vi "Calculate Best Angle.vi"(8 "Bearing Clearence":dbl, 9 "Desired Bearing":dbl, 10 "Angle (max)":dbl, 11 "Angle (min)":dbl) -> (3 "Command Heading":dbl)   [LabVIEW 2011]
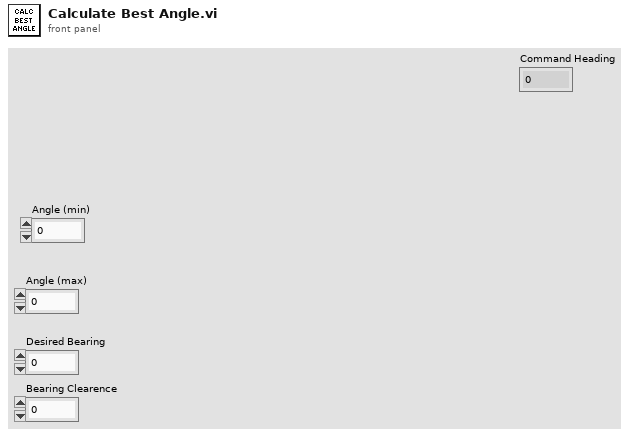
[diagram p1: front panel]
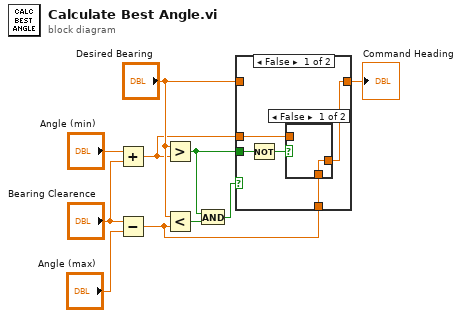
[diagram p0: block diagram]
diagram:
  n1 = Add(x="Angle (min)", y="Bearing Clearence") -> (x+y=w2:dbl)
  n2 = Subtract(x="Bearing Clearence", y="Angle (max)") -> (x-y=w1:dbl)
  n3 = Greater?(x="Desired Bearing", y=w2) -> (0:w3:bool)
  n4 = Less?(x="Desired Bearing", y=w1) -> (x < y?=w7:bool)
  n5 = And(x=w3, y=w7) -> (x .and. y?=w6:bool)
  n6 = case shown="False" w6 {
    tunnel: "Desired Bearing" -> [_ w18]
    tunnel: [w12 w18] -> w4
    tunnel: w3 -> [w15 _]
    tunnel: w2 -> [w13 _]
    tunnel: w1 -> [w11 _]
    frame False {
      n7 = Not(x=w15) -> (.not. x?=w14:bool)
      n8 = case shown="False" w14 {
        tunnel: [w16 w17] -> w12
        tunnel: w13 -> [_ w17]
        tunnel: w11 -> [w16 _]
        frame False {
        }
        frame True {
        }
      }
    }
    frame True {
    }
  }
  "Command Heading" <- w4
